vi "DashboardInterface.vi"() -> ()   [LabVIEW 2019]
uses:
  Global_Var-RefNum/AutoCommands.vi
  Global_Var-RefNum/Configurables.vi
  Global_Var-RefNum/RobotState.vi
  <vilib>/Rock Robotics/Network Tables/NT Write Boolean.vi
  <vilib>/Rock Robotics/Network Tables/NT Write Number.vi
  <vilib>/Rock Robotics/Network Tables/NT Read Number.vi
  <vilib>/Rock Robotics/Network Tables/NT Write String.vi
  Autonomous/TypeDefs/AutoMode.ctl
  <vilib>/Rock Robotics/Network Tables/NT Write String Array.vi
panel:
  in  "OldBallHoodOffsetDefault":dbl=-0.5
  in  "NewBallHoodOffsetDefault":dbl=0.5
  in  "AvgBallHoodOffsetDefault":dbl
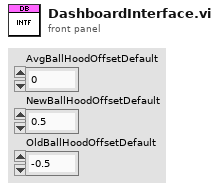
[diagram p1: front panel]
types:
  T1 = typedef "AutoMode.ctl" = enum16{"Disable", "DriveOnly", "ShootThenDrive", "DriveThenShoot", "EnemyTrench", "FriendlyTrench", "ShootThenReverse", "ReverseThenShoot"}
  T2 = typedef "ControlPanelColor.ctl" = enum16{"Blue", "Green", "Red", "Yellow", "Unknown"}
  T3 = typedef "Hood_Homing_State.ctl" = enum16{"Not Homed", "Homing in Process", "Homing Failed", "Homing Completed"}
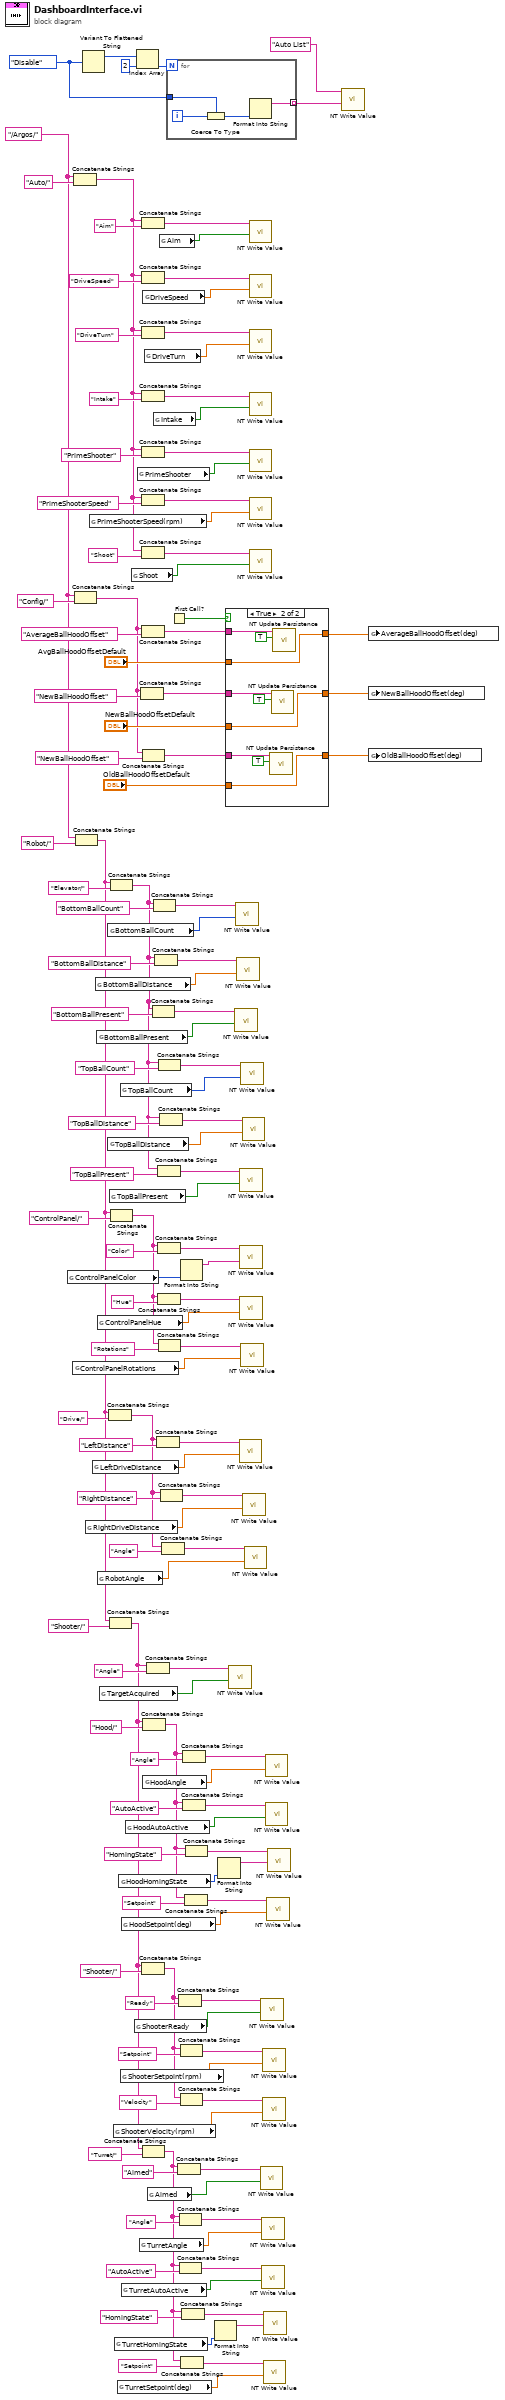
[diagram p0: block diagram]
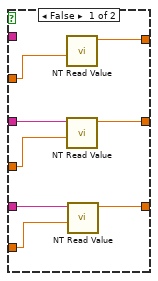
[diagram p2: hidden frame]
diagram:
  w3 = AutoMode."Disable" ("AutoMode")
  w136 = "/Argos/" ("string")
  n1 = global read "RobotState.vi" "ControlPanelColor"() -> (w65:T2)
  n2 = global read "RobotState.vi" "ControlPanelRotations"() -> (w62:dbl)
  n3 = Concatenate Strings(w136, "Auto/" ("string")) -> (w120:string)
  n4 = Concatenate Strings(w136, "Config/" ("string")) -> (w95:string)
  n5 = Concatenate Strings(w136, "Robot/" ("string")) -> (w131:string)
  n6 = Variant To Flattened String(Variant=w3) -> (1:w6:i16[])  [unwired: 1 out]
  n7 = global read "RobotState.vi" "RightDriveDistance"() -> (w53:dbl)
  n8 = global read "AutoCommands.vi" "PrimeShooterSpeed(rpm)"() -> (w107:dbl)
  n9 = global read "RobotState.vi" "LeftDriveDistance"() -> (w54:dbl)
  n10 = global read "RobotState.vi" "BottomBallDistance"() -> (w84:dbl)
  n11 = global read "RobotState.vi" "BottomBallPresent"() -> (w83:bool)
  n12 = global read "RobotState.vi" "ControlPanelHue"() -> (w63:dbl)
  n13 = global read "RobotState.vi" "RobotAngle"() -> (w52:dbl)
  n14 = global read "RobotState.vi" "TargetAcquired"() -> (w20:bool)
  n15 = global read "RobotState.vi" "BottomBallCount"() -> (w87:u16)
  n16 = global read "RobotState.vi" "TopBallDistance"() -> (w81:dbl)
  n17 = Concatenate Strings(w131, "Drive/" ("string")) -> (w55:string)
  n18 = global read "RobotState.vi" "TopBallPresent"() -> (w82:bool)
  n19 = Concatenate Strings(w131, "Shooter/" ("string")) -> (w17:string)
  n20 = Concatenate Strings(w131, "Elevator/" ("string")) -> (w73:string)
  n21 = Concatenate Strings(w131, "ControlPanel/" ("string")) -> (w67:string)
  n22 = global read "RobotState.vi" "ShooterVelocity(rpm)"() -> (w8:dbl)
  n23 = global read "RobotState.vi" "TurretHomingState"() -> (w36:T3)
  n24 = global read "RobotState.vi" "TurretSetpoint(deg)"() -> (w38:dbl)
  n25 = global read "RobotState.vi" "HoodHomingState"() -> (w41:T3)
  n26 = global read "RobotState.vi" "TopBallCount"() -> (w78:u16)
  n27 = global read "RobotState.vi" "ShooterSetpoint(rpm)"() -> (w9:dbl)
  n28 = global read "RobotState.vi" "HoodSetpoint(deg)"() -> (w39:dbl)
  n29 = global read "RobotState.vi" "TurretAutoActive"() -> (w34:bool)
  n30 = global read "RobotState.vi" "HoodAutoActive"() -> (w43:bool)
  n31 = global read "AutoCommands.vi" "Shoot"() -> (w106:bool)
  n32 = global read "RobotState.vi" "ShooterReady"() -> (w16:bool)
  n33 = Index Array(array=w6, index=2) -> (element=w4:i16)
  n34 = global read "AutoCommands.vi" "PrimeShooter"() -> (w108:bool)
  n35 = global read "RobotState.vi" "TurretAngle"() -> (w33:dbl)
  n36 = Concatenate Strings(w95, "NewBallHoodOffset" ("string")) -> (w99:string)
  n37 = Concatenate Strings(w120, "Aim" ("string")) -> (w119:string)
  n38 = Concatenate Strings(w120, "DriveSpeed" ("string")) -> (w118:string)
  n39 = Concatenate Strings(w120, "DriveTurn" ("string")) -> (w117:string)
  n40 = Concatenate Strings(w120, "Intake" ("string")) -> (w116:string)
  n41 = Concatenate Strings(w120, "PrimeShooter" ("string")) -> (w115:string)
  n42 = Concatenate Strings(w120, "PrimeShooterSpeed" ("string")) -> (w114:string)
  n43 = Concatenate Strings(w120, "Shoot" ("string")) -> (w113:string)
  n44 = Concatenate Strings(w95, "AverageBallHoodOffset" ("string")) -> (w104:string)
  n45 = Concatenate Strings(w17, "Shooter/" ("string")) -> (w7:string)
  n46 = Concatenate Strings(w95, "NewBallHoodOffset" ("string")) -> (w94:string)
  n47 = Concatenate Strings(w17, "Turret/" ("string")) -> (w22:string)
  n48 = global read "AutoCommands.vi" "DriveSpeed"() -> (w111:dbl)
  n49 = Concatenate Strings(w17, "Hood/" ("string")) -> (w21:string)
  n50 = global read "RobotState.vi" "HoodAngle"() -> (w44:dbl)
  n51 = global read "AutoCommands.vi" "DriveTurn"() -> (w110:dbl)
  n52 = Concatenate Strings(w17, "Angle" ("string")) -> (w19:string)
  n53 = global read "RobotState.vi" "Aimed"() -> (w23:bool)
  n54 = Concatenate Strings(w73, "BottomBallPresent" ("string")) -> (w86:string)
  n55 = global read "AutoCommands.vi" "Intake"() -> (w109:bool)
  n56 = Concatenate Strings(w73, "BottomBallCount" ("string")) -> (w90:string)
  n57 = Concatenate Strings(w73, "BottomBallDistance" ("string")) -> (w88:string)
  n58 = Concatenate Strings(w55, "LeftDistance" ("string")) -> (w61:string)
  n59 = Concatenate Strings(w73, "TopBallPresent" ("string")) -> (w79:string)
  n60 = Concatenate Strings(w67, "Color" ("string")) -> (w66:string)
  n61 = Concatenate Strings(w67, "Hue" ("string")) -> (w69:string)
  n62 = Concatenate Strings(w73, "TopBallCount" ("string")) -> (w75:string)
  n63 = Concatenate Strings(w67, "Rotations" ("string")) -> (w68:string)
  n64 = global read "AutoCommands.vi" "Aim"() -> (w112:bool)
  n65 = Concatenate Strings(w73, "TopBallDistance" ("string")) -> (w77:string)
  n66 = Concatenate Strings(w55, "RightDistance" ("string")) -> (w58:string)
  n67 = Concatenate Strings(w55, "Angle" ("string")) -> (w57:string)
  n68 = for {
    N: w4 -> [_]
    tunnel: w3 -> [w142]
    tunnel: [w140] -> w2 mode=indexing
    i -> [w143]
    n69 = Coerce To Type(0:w143, 1:w142) -> (2:w141:T1)
    n70 = Format Into String(w141) -> (resulting string=w140:string)  [unwired: 3 in, 1 out]
  }
  n71 = First Call?() -> (First Call?: T/F=w103:bool)
  n72 = Concatenate Strings(w22, "Aimed" ("string")) -> (w24:string)
  n73 = Concatenate Strings(w7, "Ready" ("string")) -> (w15:string)
  n74 = Concatenate Strings(w22, "Angle" ("string")) -> (w27:string)
  n75 = Concatenate Strings(w22, "AutoActive" ("string")) -> (w28:string)
  n76 = Format Into String(w65) -> (resulting string=w64:string)  [unwired: 3 in, 1 out]
  n77 = Concatenate Strings(w7, "Setpoint" ("string")) -> (w12:string)
  n78 = Concatenate Strings(w7, "Velocity" ("string")) -> (w11:string)
  n79 = Concatenate Strings(w22, "Setpoint" ("string")) -> (w31:string)
  n80 = Concatenate Strings(w22, "HomingState" ("string")) -> (w35:string)
  n81 = Concatenate Strings(w21, "Angle" ("string")) -> (w50:string)
  n82 = Concatenate Strings(w21, "AutoActive" ("string")) -> (w49:string)
  n83 = Concatenate Strings(w21, "Setpoint" ("string")) -> (w46:string)
  n84 = Concatenate Strings(w21, "HomingState" ("string")) -> (w42:string)
  n85 = Format Into String(w36) -> (resulting string=w37:string)  [unwired: 3 in, 1 out]
  n86 = Format Into String(w41) -> (resulting string=w40:string)  [unwired: 3 in, 1 out]
  n87 = case shown="True" w103 {
    tunnel: w104 -> [_ w159]
    tunnel: [w151 w158] -> w102
    tunnel: "AvgBallHoodOffsetDefault" -> [w150 w158]
    tunnel: w99 -> [w149 w156]
    tunnel: [w148 w155] -> w98
    tunnel: "NewBallHoodOffsetDefault" -> [w147 w155]
    tunnel: w94 -> [w146 w153]
    tunnel: [w145 w152] -> w93
    tunnel: "OldBallHoodOffsetDefault" -> [w144 w152]
    frame False {
      n88 = call-poly <vilib>:"NT Read Value.vi"("Default Value"=w150) -> ("Numeric"=w151:dbl)  [unwired: 9 in, 1 out]
      n89 = call-poly <vilib>:"NT Read Value.vi"("Default Value"=w147, "Name"=w149) -> ("Numeric"=w148:dbl)  [unwired: 8 in, 1 out]
      n90 = call-poly <vilib>:"NT Read Value.vi"("Default Value"=w144, "Name"=w146) -> ("Numeric"=w145:dbl)  [unwired: 8 in, 1 out]
    }
    frame True {
      n91 = call <vilib>:"NT Update Persistence.vi"("Persistence"=TRUE, "Name"=w153) -> ()  [unwired: 9 in, 1 out]
      n92 = call <vilib>:"NT Update Persistence.vi"("Persistence"=TRUE, "Name"=w156) -> ()  [unwired: 9 in, 1 out]
      n93 = call <vilib>:"NT Update Persistence.vi"("Persistence"=TRUE, "Name"=w159) -> ()  [unwired: 9 in, 1 out]
    }
  }
  n94 = call-poly <vilib>:"NT Write Value.vi"("Boolean"=w20, "Name"=w19) -> ()  [unwired: 9 in, 1 out]
  n95 = call-poly <vilib>:"NT Write Value.vi"("Boolean"=w83, "Name"=w86) -> ()  [unwired: 9 in, 1 out]
  n96 = call-poly <vilib>:"NT Write Value.vi"("Numeric"=w87, "Name"=w90) -> ()  [unwired: 9 in, 1 out]
  n97 = call-poly <vilib>:"NT Write Value.vi"("Numeric"=w84, "Name"=w88) -> ()  [unwired: 9 in, 1 out]
  n98 = call-poly <vilib>:"NT Write Value.vi"("Numeric"=w54, "Name"=w61) -> ()  [unwired: 9 in, 1 out]
  n99 = call-poly <vilib>:"NT Write Value.vi"("Boolean"=w82, "Name"=w79) -> ()  [unwired: 9 in, 1 out]
  n100 = call-poly <vilib>:"NT Write Value.vi"("String"=w64, "Name"=w66) -> ()  [unwired: 9 in, 1 out]
  n101 = call-poly <vilib>:"NT Write Value.vi"("Numeric"=w63, "Name"=w69) -> ()  [unwired: 9 in, 1 out]
  n102 = call-poly <vilib>:"NT Write Value.vi"("Numeric"=w78, "Name"=w75) -> ()  [unwired: 9 in, 1 out]
  n103 = call-poly <vilib>:"NT Write Value.vi"("Numeric"=w62, "Name"=w68) -> ()  [unwired: 9 in, 1 out]
  n104 = call-poly <vilib>:"NT Write Value.vi"("Numeric"=w81, "Name"=w77) -> ()  [unwired: 9 in, 1 out]
  n105 = call-poly <vilib>:"NT Write Value.vi"("Numeric"=w53, "Name"=w58) -> ()  [unwired: 9 in, 1 out]
  n106 = call-poly <vilib>:"NT Write Value.vi"("Numeric"=w52, "Name"=w57) -> ()  [unwired: 9 in, 1 out]
  n107 = call-poly <vilib>:"NT Write Value.vi"("Boolean"=w112, "Name"=w119) -> ()  [unwired: 9 in, 1 out]
  n108 = call-poly <vilib>:"NT Write Value.vi"("Numeric"=w111, "Name"=w118) -> ()  [unwired: 9 in, 1 out]
  n109 = call-poly <vilib>:"NT Write Value.vi"("Numeric"=w110, "Name"=w117) -> ()  [unwired: 9 in, 1 out]
  n110 = call-poly <vilib>:"NT Write Value.vi"("Boolean"=w109, "Name"=w116) -> ()  [unwired: 9 in, 1 out]
  n111 = call-poly <vilib>:"NT Write Value.vi"("Boolean"=w108, "Name"=w115) -> ()  [unwired: 9 in, 1 out]
  n112 = call-poly <vilib>:"NT Write Value.vi"("Numeric"=w107, "Name"=w114) -> ()  [unwired: 9 in, 1 out]
  n113 = call-poly <vilib>:"NT Write Value.vi"("Boolean"=w106, "Name"=w113) -> ()  [unwired: 9 in, 1 out]
  n114 = call-poly <vilib>:"NT Write Value.vi"("Boolean"=w23, "Name"=w24) -> ()  [unwired: 9 in, 1 out]
  n115 = call-poly <vilib>:"NT Write Value.vi"("Boolean"=w16, "Name"=w15) -> ()  [unwired: 9 in, 1 out]
  n116 = call-poly <vilib>:"NT Write Value.vi"("Numeric"=w33, "Name"=w27) -> ()  [unwired: 9 in, 1 out]
  n117 = call-poly <vilib>:"NT Write Value.vi"("Boolean"=w34, "Name"=w28) -> ()  [unwired: 9 in, 1 out]
  n118 = call-poly <vilib>:"NT Write Value.vi"("Numeric"=w9, "Name"=w12) -> ()  [unwired: 9 in, 1 out]
  n119 = call-poly <vilib>:"NT Write Value.vi"("Numeric"=w8, "Name"=w11) -> ()  [unwired: 9 in, 1 out]
  n120 = call-poly <vilib>:"NT Write Value.vi"("Numeric"=w38, "Name"=w31) -> ()  [unwired: 9 in, 1 out]
  n121 = call-poly <vilib>:"NT Write Value.vi"("String"=w37, "Name"=w35) -> ()  [unwired: 9 in, 1 out]
  n122 = call-poly <vilib>:"NT Write Value.vi"("Numeric"=w44, "Name"=w50) -> ()  [unwired: 9 in, 1 out]
  n123 = call-poly <vilib>:"NT Write Value.vi"("Boolean"=w43, "Name"=w49) -> ()  [unwired: 9 in, 1 out]
  n124 = call-poly <vilib>:"NT Write Value.vi"("Numeric"=w39, "Name"=w46) -> ()  [unwired: 9 in, 1 out]
  n125 = call-poly <vilib>:"NT Write Value.vi"("String"=w40, "Name"=w42) -> ()  [unwired: 9 in, 1 out]
  n126 = call-poly <vilib>:"NT Write Value.vi"("String Array"=w2, "Name"="Auto List") -> ()  [unwired: 9 in, 1 out]
  n127 = global write "Configurables.vi" "AverageBallHoodOffset(deg)"(w102) -> ()
  n128 = global write "Configurables.vi" "NewBallHoodOffset(deg)"(w98) -> ()
  n129 = global write "Configurables.vi" "OldBallHoodOffset(deg)"(w93) -> ()
